vi "Launch Meter Actor.vi"(8 "error in":errorcluster, 11 "SCADA in":refnum<class "EMS.lvclass">) -> (0 "error out":errorcluster, 3 "SCADA out":refnum<class "EMS.lvclass">)   [LabVIEW 2018, in "EMS Core.lvlib" / "EMS.lvclass"]
uses:
  EMS.lvclass
  C:/Users/Administrator/Desktop/LabVIEW EMS/EMS Generic Actor/EMS Generic/EMS Generic.lvclass
  C:/Program Files (x86)/National Instruments/LabVIEW 2018/vi.lib/ActorFramework/Actor/Actor.lvclass
  IED Actors/Meter Actor/Meter/Meter.lvclass
  <vilib>/ORNL/CSEISMIC DDS/CSEISMIC DDS Base/Data Types/Controls/DeviceClass Selector.ctl
  EMS.lvclass/EMS.ctl
  <vilib>/ActorFramework/Actor/Actor.lvclass
  <vilib>/ORNL/CSEISMIC DDS/CSEISMIC DDS Base/CSEISMIC DDS.lvclass
  EMS Generic Actor/EMS Generic/EMS Generic.lvclass
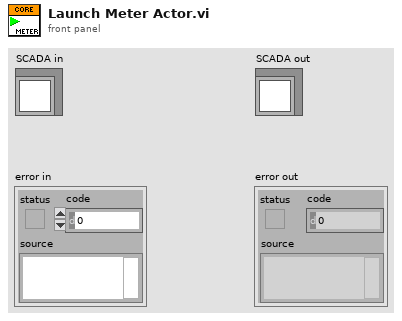
[diagram p1: front panel]
types:
  T1 = typedef "CSEISMIC DDS.lvlib/CSEISMIC DDS.lvclass/DeviceID.ctl" = string
  T2 = typedef "CSEISMIC DDS.lvlib/CSEISMIC DDS.lvclass/DeviceClass Selector.ctl" = u16
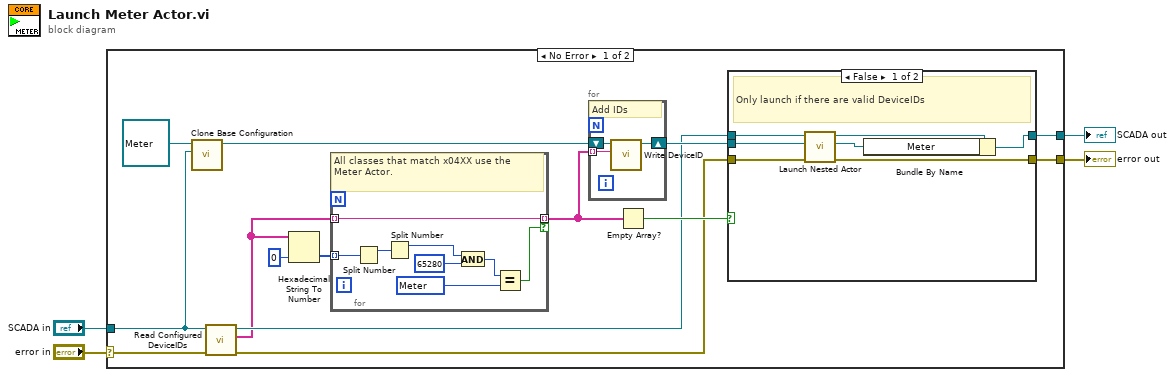
[diagram p0: block diagram]
diagram:
  n1 = case shown="No Error" "error in" {
    selector: "error in" -> [w8 w40]
    tunnel: [w17 w40] -> w3
    tunnel: [w18 w39] -> w1
    tunnel: "SCADA in" -> [w5 w39]
    frame No Error {
      n2 = call-dynamic "Clone Base Configuration.vi"("Source Object"=w5, "Target Object in"=refnum<class "Meter.lvclass"> refnum ("Meter Actor.lvlib:Meter.lvclass")) -> ("Target Object out"=w6:refnum<class "Meter.lvclass">)  [unwired: 9 in]
      n3 = call "Read Configured DeviceIDs.vi"("error in"=w8, "EMS Generic in"=w5) -> ("error out"=w13:errorcluster, "DeviceIDs"=w11:T1[], "EMS Generic out"=w12:refnum<class "EMS.lvclass">)  [unwired: 7 in]
      n4 = Hexadecimal String To Number(string=w11, default (0uL)=u64 0 ("default (0 U32)")) -> (number=w9:u64[])  [unwired: 1 in, 1 out]
      n5 = for {
        tunnel: w11 -> [w28] mode=indexing
        tunnel: [w28] -> w15 mode=indexing if=w27
        tunnel: w9 -> [w22] mode=indexing
        w26 = T2 1024 items=["Invalid"=0, "IED"=256, "DER"=512, "Relay"=768, "Meter"=1024, "Load"=1280, "Energy Storage"=513, "PV"=514, "Generator"=515, "Smart Relay"=769, "PCC"=770, "Smart Meter"=1025, "PMU"=1026, "HVAC"=1281] ("DeviceClass")
        # "All classes that match x04XX use the Meter Actor."
        n6 = Split Number(x=w22) -> (hi(x)=w29:u32)  [unwired: 1 out]
        n7 = Split Number(x=w29) -> (hi(x)=w25:u16)  [unwired: 1 out]
        n8 = And(x=w25, y=u16 65280) -> (x .and. y?=w24:u16)
        n9 = Equal?(x=w24, y=w26) -> (x = y?=w27:bool)
      }
      n10 = for {
        shift-right: [w20] -> w16
        shift-left: w6 -> [w21]
        tunnel: w15 -> [w19] mode=indexing
        # "Add IDs"
        n11 = call-dynamic "Write DeviceID.vi"("DeviceID"=w19, "Device DDS Communications in"=w21) -> ("Device DDS Communications out"=w20:refnum<class "Meter.lvclass">)  [unwired: 9 in]
      }
      n12 = Empty Array?(array=w15) -> (empty?=w14:bool)
      n13 = case shown="False" w14 {
        tunnel: [w31 w38] -> w18
        tunnel: w13 -> [w35 w37]
        tunnel: [w34 w37] -> w17
        tunnel: w16 -> [w33 _]
        tunnel: w12 -> [w32 w38]
        frame False {
          # "Only launch if there are valid DeviceIDs"
          n14 = call <vilib>:"Launch Nested Actor.vi"("error in (no error)"=w35, "Nested Actor"=w33, "Caller Actor in"=w32) -> ("error out"=w34:errorcluster, "Nested Actor's Enqueuer"=w30:refnum<class "Message Enqueuer.lvclass">, "Caller Actor out"=w36:refnum<class "EMS.lvclass">)  [unwired: 6 in]
          n15 = Bundle By Name(cluster=w36, "Meter"=w30) -> (w31:refnum<class "EMS.lvclass">)
        }
        frame True {
        }
      }
    }
    frame Error {
    }
  }
  "error out" <- w3
  "SCADA out" <- w1
